vi "Demo3-网页内的对象控制与交互之表格.vi"() -> ()   [LabVIEW 2011]
panel:
  out "每行单元格数":i32
  out "获取单元格内容":string
  out "取出一行内容":string
  out "行数":i32
  out "outerText":string
  out "outerHTML":string
  in  "WebBrowser":refnum<k7>(container)
  in  "htmlDoc3":refnum<k7>
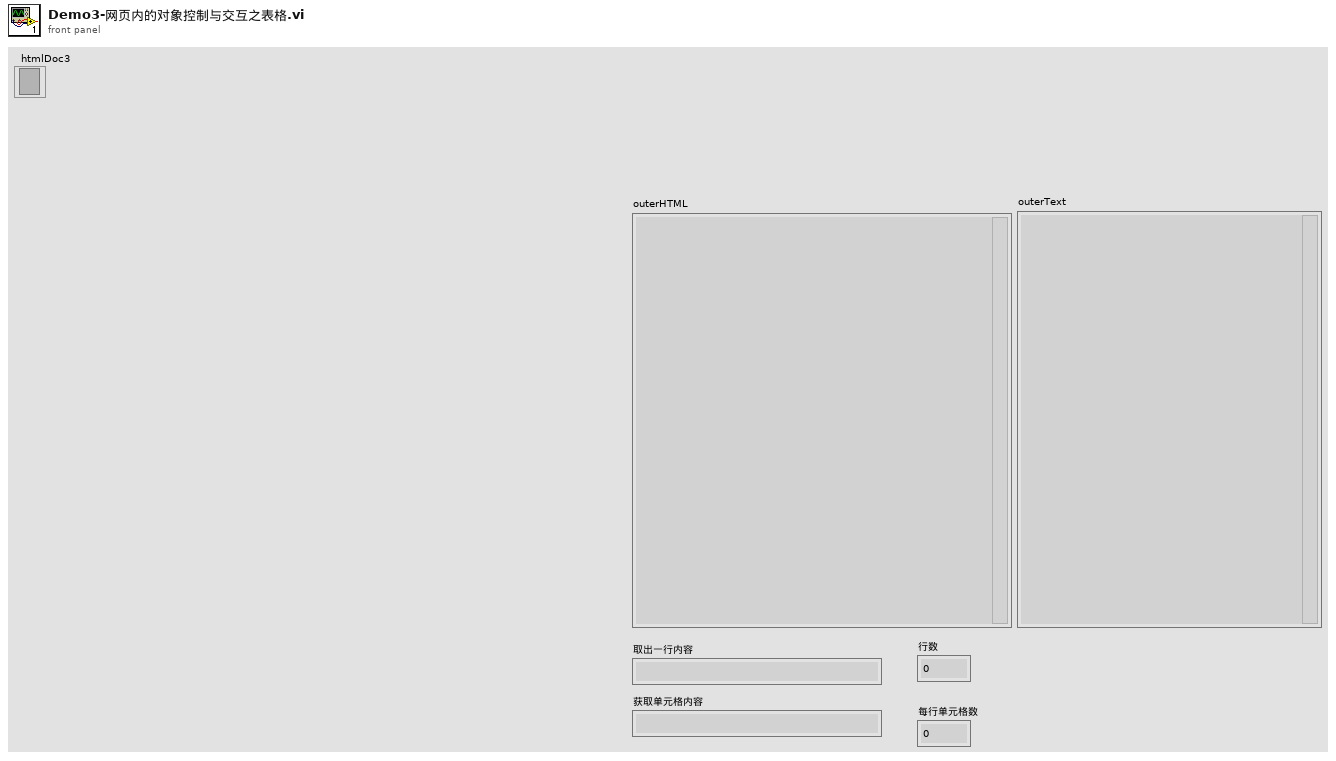
[diagram p1: front panel]
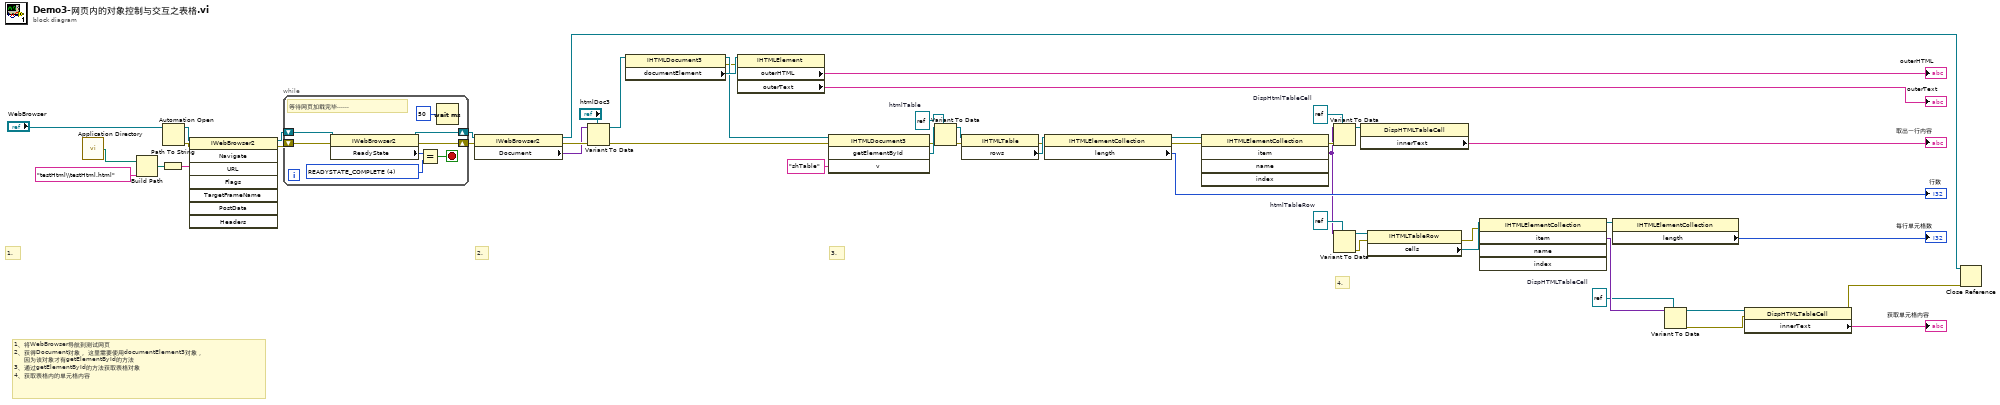
[diagram p0: block diagram]
diagram:
  w21 = refnum<k7> refnum  # DispHTMLTableCell
  w27 = refnum<k7> refnum  # DispHtmlTableCell
  w24 = refnum<k7> refnum  # htmlTableRow
  w33 = refnum<k7> refnum  # htmlTable
  # "1、将WebBrowser导航到测试网页\n2、获得Document对象， 这里需要使用documentElement3对象，\n     因为该对象才有getElementById的方法\n3、通过getElementById的方法获取表格对象\n4、获取表格内的单元格内容"
  # "4."
  # "3."
  # "2."
  # "1."
  n1 = call <vilib>:"Application Directory.vi"() -> ("Application Directory"=w1:path)
  n2 = Build Path(base path=w1, name or relative path="testHtml\\testHtml.html" ("名称或相对路径")) -> (appended path=w38:path)
  n3 = Path To String(path=w38) -> (string=w34:string)
  n4 = Automation Open(Automation Refnum="WebBrowser") -> (Automation Refnum=w44:refnum<k7>, error out=w45:errorcluster)  [unwired: 3 in]
  n5 = invoke class="IWebBrowser2" method="Navigate"(reference=w44, error in=w45, "URL"=w34) -> (reference out=w49:refnum<k7>, error out=w47:errorcluster)  [unwired: 5 in, 6 out]
  n6 = while {
    shift-right: [w59] -> w48
    shift-left: w49 -> [w52]
    shift-right: [w53] -> w46
    shift-left: w47 -> [w54]
    stop <- w56 stop-if-true
    w58 = 4 items=["READYSTATE_UNINITIALIZED", "READYSTATE_LOADING", "READYSTATE_LOADED", "READYSTATE_INTERACTIVE", "READYSTATE_COMPLETE"] ("ReadyState")
    # "等待网页加载完毕......"
    n7 = property class="IWebBrowser2"(reference=w52, error in=w54) -> (reference out=w59:refnum<k7>, error out=w53:errorcluster, "ReadyState"=w57:i32)
    n8 = Equal?(x=w57, y=w58) -> (x = y?=w56:bool)
    n9 = Wait (ms)(milliseconds to wait=u32 50 ("等待时间（毫秒）")) -> ()  [unwired: 1 out]
  }
  n10 = property class="IWebBrowser2"(reference=w48, error in=w46) -> (reference out=w3:refnum<k7>, error out=w51:errorcluster, "Document"=w43:variant)
  n11 = Variant To Data(error in=w51, type="htmlDoc3", Variant=w43) -> (data=w7:refnum<k7>, error out=w41:errorcluster)
  n12 = property class="IHTMLDocument3"(reference=w7) -> (reference out=w6:refnum<k7>, error out=w5:errorcluster, "documentElement"=w37:refnum<k7>)  [unwired: 1 in]
  n13 = property class="IHTMLElement"(reference=w37, error in=w5) -> ("outerHTML"=→"outerHTML":string, "outerText"=→"outerText":string)  [unwired: 2 out]
  n14 = invoke class="IHTMLDocument3" method="getElementById"(reference=w6, error in=w41, "v"="shTable") -> (error out=w11:errorcluster, "getElementById"=w40:refnum<k7>)  [unwired: 1 in, 2 out]
  n15 = Variant To Data(error in=w11, type=w33, Variant=w40) -> (data=w31:refnum<k7>, error out=w12:errorcluster)
  n16 = property class="IHTMLTable"(reference=w31, error in=w12) -> (error out=w13:errorcluster, "rows"=w30:refnum<k7>)  [unwired: 1 out]
  n17 = property class="IHTMLElementCollection"(reference=w30, error in=w13) -> (reference out=w14:refnum<k7>, error out=w9:errorcluster, "length"=→"行数":i32)
  n18 = invoke class="IHTMLElementCollection" method="item"(reference=w14, error in=w9) -> (error out=w29:errorcluster, "item"=w10:variant)  [unwired: 3 in, 3 out]
  n19 = Variant To Data(error in=w29, type=w27, Variant=w10) -> (data=w25:refnum<k7>)  [unwired: 1 out]
  n20 = Variant To Data(type=w24, Variant=w10) -> (data=w23:refnum<k7>, error out=w15:errorcluster)  [unwired: 1 in]
  n21 = property class="DispHTMLTableCell"(reference=w25) -> ("innerText"=→"取出一行内容":string)  [unwired: 1 in, 2 out]
  n22 = property class="IHTMLTableRow"(reference=w23, error in=w15) -> (error out=w16:errorcluster, "cells"=w26:refnum<k7>)  [unwired: 1 out]
  n23 = invoke class="IHTMLElementCollection" method="item"(reference=w26, error in=w16) -> (reference out=w8:refnum<k7>, "item"=w22:variant)  [unwired: 3 in, 3 out]
  n24 = property class="IHTMLElementCollection"(reference=w8) -> ("length"=→"每行单元格数":i32)  [unwired: 1 in, 2 out]
  n25 = Variant To Data(type=w21, Variant=w22) -> (data=w20:refnum<k7>, error out=w19:errorcluster)  [unwired: 1 in]
  n26 = property class="DispHTMLTableCell"(reference=w20, error in=w19) -> (error out=w4:errorcluster, "innerText"=→"获取单元格内容":string)  [unwired: 1 out]
  n27 = Close Reference(reference=w3, error in (no error)=w4) -> ()  [unwired: 1 out]
